vi "Position measurement.vi"(1 "Measure \nintensities":bool, 3 "ROI size":dbl=20.0, 5 "Acquired Buffer Number":u32, 6 "Switch xy":bool, 7 "Coordinate mapping \n(Monitor to Measurement)":T1, 8 "ROIs":T2[](array[typedef]), 9 "Target positions (monitor)":T3, 10 "Image":T2) -> (0 "Target coordinates (measurement)":cluster{"X target":sgl[], "Y target":sgl[]}, 2 "Position data out (measurement)":T4)   [LabVIEW 2012]
uses:
  Trap cluster.ctl
  <vilib>/vision/Image Controls.llb/IMAQ Image.ctl
  <vilib>/vision/NI_Vision_Development_Module.lvlib
panel:
  in  "Display ROI nr":i32
  out "Image 2":T2(plugin-control)
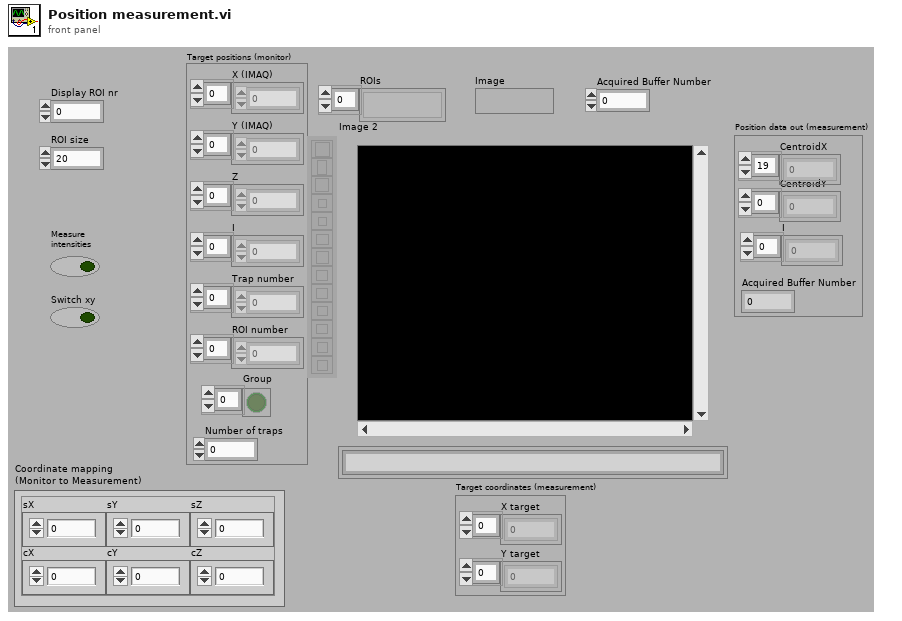
[diagram p1: front panel]
types:
  T1 = cluster{"cZ":sgl, "cY":sgl, "cX":sgl, "sZ":sgl, "sY":sgl, "sX":sgl}
  T2 = typedef "IMAQ Image.ctl" = refnum<image>
  T3 = typedef "Trap cluster.ctl" = cluster{"X (IMAQ)":sgl[], "Y (IMAQ)":sgl[], "Z":sgl[], "I":sgl[], "Trap number":i32[], "ROI number":i32[], "Number of traps":i32, "Group":bool[]}
  T4 = cluster{"CentroidX":dbl[], "CentroidY":dbl[], "I":dbl[], "Acquired Buffer Number":u32}
  T5 = cluster{"X (Measurement)":sgl[], "Y (Measurement)":sgl[]}
  T6 = cluster{dbl[], dbl[], dbl[], "Acquired Buffer Number":u32}
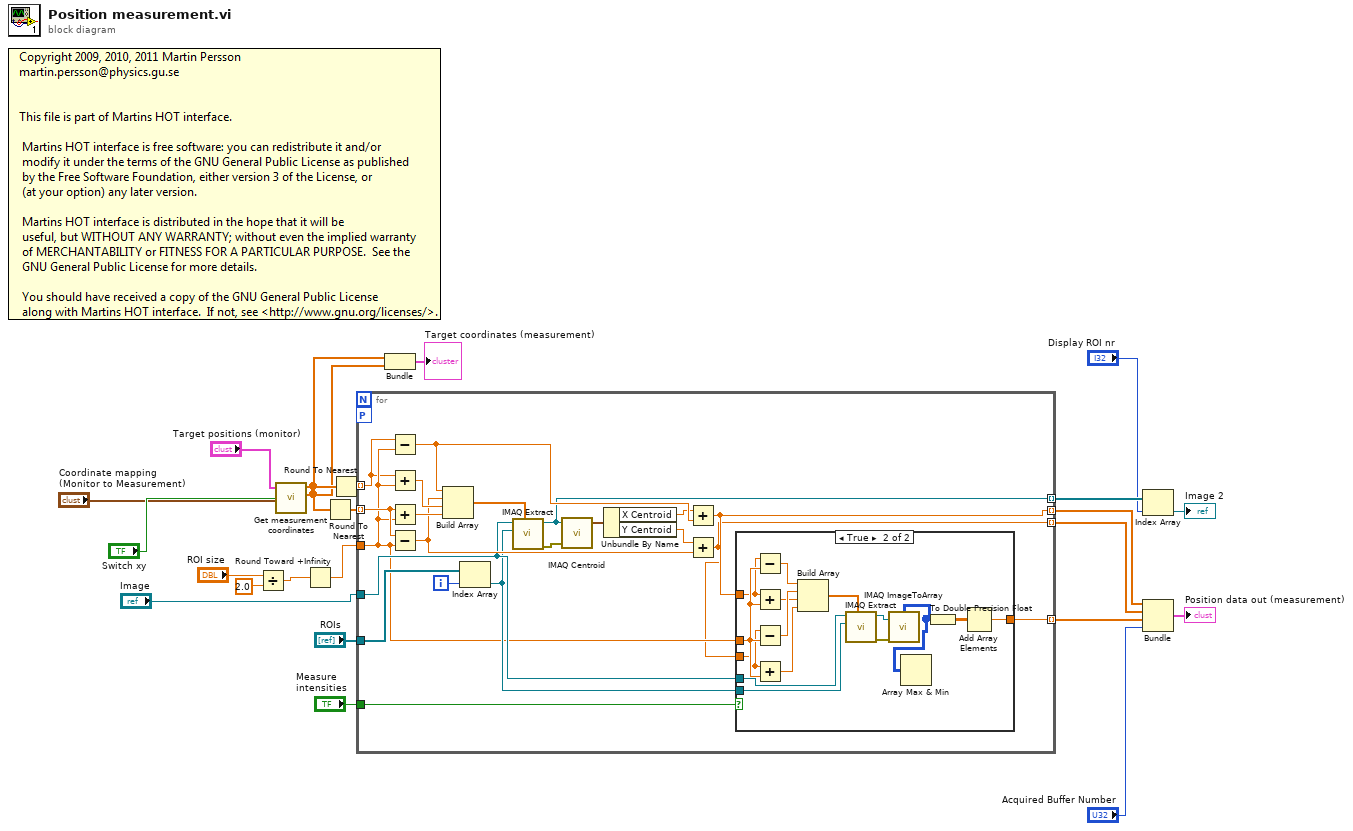
[diagram p0: block diagram]
diagram:
  n1 = Divide(x="ROI size", y=2.0) -> (x/y=w22:dbl)
  n2 = call "Get measurement coordinates.vi"("Trap cluster"="Target positions (monitor)", "Switch xy"="Switch xy", "Coordinate mapping \n(Monitor to Measurement)"="Coordinate mapping \n(Monitor to Measurement)") -> ("X (Measurement)"=w5:sgl[], "Y (Measurement)"=w4:sgl[])  [unwired: 3 in]
  n3 = Round Toward +Infinity(x=w22) -> (ceil(x): smallest int >= x=w16:dbl)
  n4 = Round To Nearest(number=w4) -> (nearest integer value=w1:sgl[])
  n5 = Round To Nearest(number=w5) -> (nearest integer value=w2:sgl[])
  n6 = for {
    tunnel: w1 -> [w43] mode=indexing
    tunnel: "Image" -> [w31]
    tunnel: "ROIs" -> [w44]
    tunnel: w16 -> [w29]
    tunnel: [w26] -> w11 mode=indexing
    tunnel: [w25] -> w10 mode=indexing
    tunnel: [w33] -> w20 mode=indexing
    workers-P: _ -> [_]
    tunnel: [w32] -> w14 mode=indexing
    tunnel: "Measure \nintensities" -> [w27]
    tunnel: w2 -> [w24] mode=indexing
    i -> [w34]
    n7 = Subtract(x=w24, y=w29) -> (x-y=w37:dbl)
    n8 = Add(x=w24, y=w29) -> (x+y=w42:dbl)
    n9 = Add(x=w43, y=w29) -> (x+y=w41:dbl)
    n10 = Subtract(x=w43, y=w29) -> (x-y=w35:dbl)
    n11 = Build Array(w37, w35, w42, w41) -> (w40:dbl[])
    n12 = Index Array(array=w44, index=w34) -> (element=w30:T2)
    n13 = call "IMAQ Extract"("Optional Rectangle"=w40, "Image Dst"=w30, "Image Src"=w31) -> ("error out"=w39:errorcluster, "Image Dst Out"=w33:T2)  [unwired: 7 in]
    n14 = call "IMAQ Centroid"("error in (no error)"=w39, "Image"=w33) -> ("Centroid"=w38:cluster{"X Centroid":sgl, "Y Centroid":sgl})  [unwired: 2 in, 1 out]
    n15 = Unbundle By Name(w38) -> ("X Centroid"=w36:sgl, "Y Centroid"=w28:sgl)
    n16 = Add(x=w36, y=w37) -> (x+y=w26:dbl)
    n17 = Add(x=w28, y=w35) -> (x+y=w25:dbl)
    n18 = case shown="True" w27 {
      tunnel: [_ w46] -> w32
      tunnel: w31 -> [_ w52]
      tunnel: w30 -> [_ w59]
      tunnel: w29 -> [_ w58]
      tunnel: w26 -> [_ w57]
      tunnel: w25 -> [_ w47]
      frame False {
      }
      frame True {
        n19 = Subtract(x=w57, y=w58) -> (x-y=w51:dbl)
        n20 = Add(x=w57, y=w58) -> (x+y=w49:dbl)
        n21 = Subtract(x=w47, y=w58) -> (x-y=w50:dbl)
        n22 = Add(x=w47, y=w58) -> (x+y=w48:dbl)
        n23 = Build Array(w51, w50, w49, w48) -> (w53:dbl[])
        n24 = call "IMAQ Extract"("Optional Rectangle"=w53, "Image Dst"=w59, "Image Src"=w52) -> ("error out"=w55:errorcluster, "Image Dst Out"=w54:T2)  [unwired: 7 in]
        n25 = call "IMAQ ImageToArray"("error in (no error)"=w55, "Image"=w54) -> ("Image Pixels (U8)"=w45:u8[][])  [unwired: 2 in, 4 out]
        n26 = Array Max & Min(array=w45) -> ()  [unwired: 4 out]
        n27 = To Double Precision Float(number=w45) -> (double precision float=w56:dbl[][])
        n28 = Add Array Elements(numeric array=w56) -> (sum=w46:dbl)
      }
    }
  }
  n29 = Bundle("X (Measurement)"=w5, "Y (Measurement)"=w4) -> (→"Target coordinates (measurement)":T5)  [unwired: 1 in]
  n30 = Index Array(array=w20, index="Display ROI nr") -> (element=→"Image 2":T2)
  n31 = Bundle(w11, w10, w14, "Acquired Buffer Number"="Acquired Buffer Number") -> (→"Position data out (measurement)":T6)  [unwired: 1 in]
